vi "CombineVIScreenshots.vi"(6 "Image Types":T1[](array[typedef]), 8 "error in (no error)":errorcluster, 9 "Output Folders":T5, 10 "NewVI Screenshots in":T2, 11 "OldVI Screenshots in":T2) -> (0 "error out":errorcluster)   [LabVIEW 2015, in "VIDiffScreenshots.lvlib"]
uses:
  VIDiffScreenshots.lvlib
  Utilities/Output Folders.ctl
  VIScreenshots.ctl
  ScreenshotInfo.ctl
  Screenshot Type.ctl
  Utilities/FilePaths.ctl
  Utilities/VIDiffUtilities.lvlib
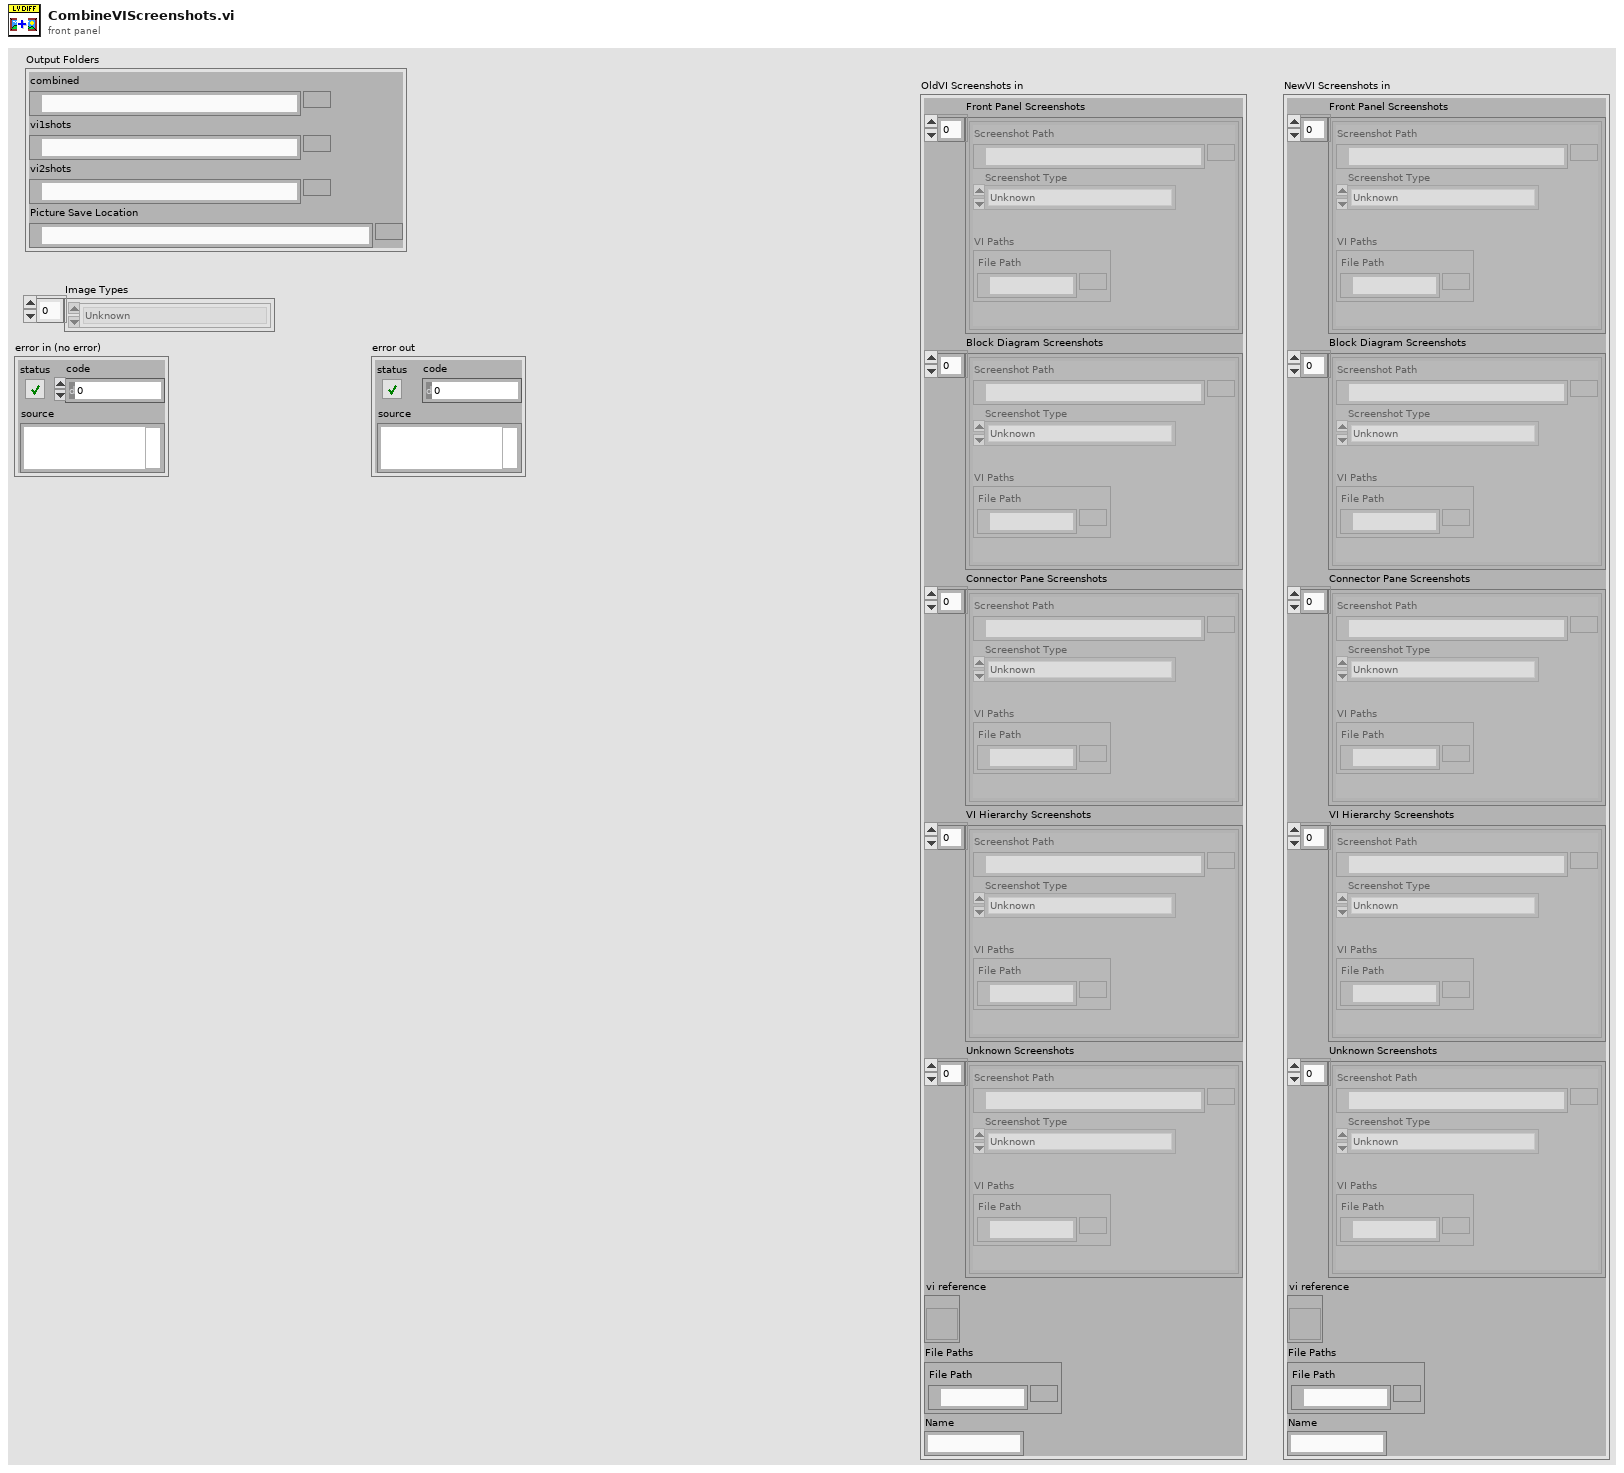
[diagram p1: front panel]
types:
  T1 = typedef "VIDiffScreenshots.lvlib/Screenshot Type.ctl" = enum16{"Unknown", "Front Panel", "Connector Pane", "Block Diagram", "VI Hierarchy"}
  T2 = typedef "VIDiffScreenshots.lvlib/VIScreenshots.ctl" = cluster{"Front Panel Screenshots":T3[], "Block Diagram Screenshots":T3[], "Connector Pane Screenshots":T3[], "VI Hierarchy Screenshots":T3[], "Unknown Screenshots":T3[], "vi reference":refnum<vi>, "File Paths":cluster{"File Path":path}, "Name":string}
  T3 = typedef "VIDiffScreenshots.lvlib/ScreenshotInfo.ctl" = cluster{"Screenshot Path":path, "Screenshot Type":T1, "VI Paths":T4}
  T4 = typedef "VIDiffUtilities.lvlib/FilePaths.ctl" = cluster{"File Path":path}
  T5 = typedef "VIDiffUtilities.lvlib/Output Folders.ctl" = cluster{"combined":path, "vi1shots":path, "vi2shots":path, "Picture Save Location":path}
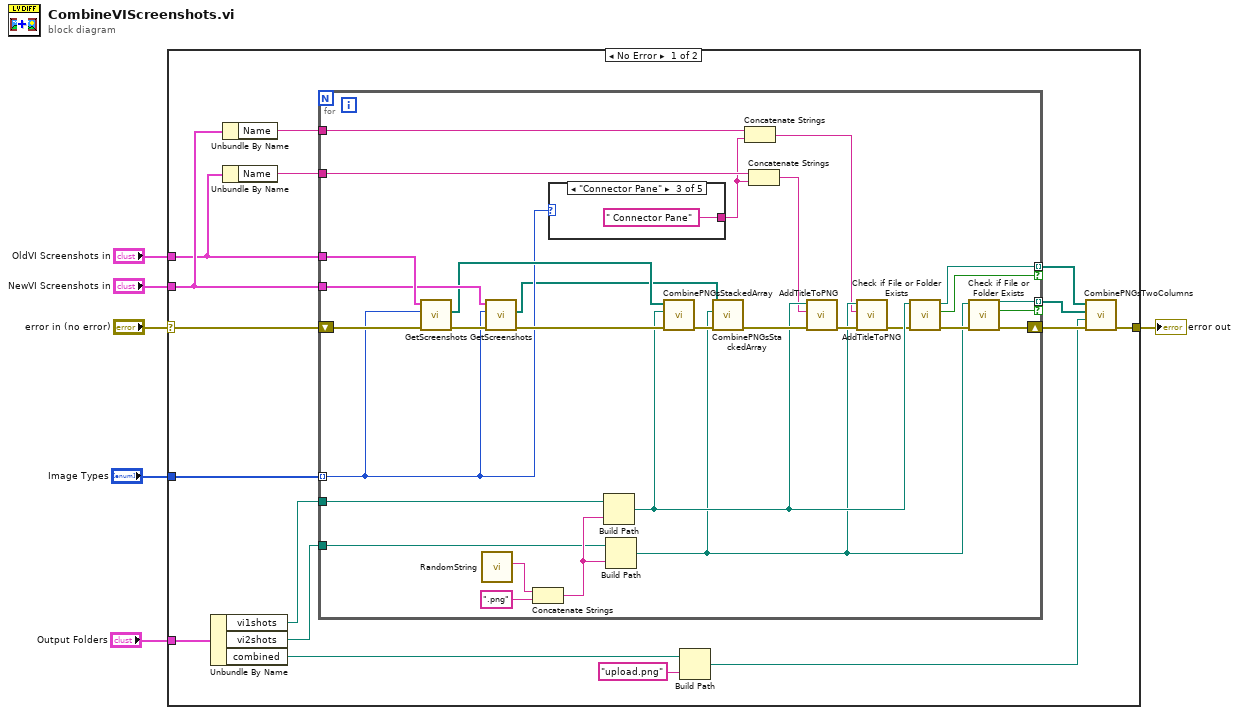
[diagram p0: block diagram]
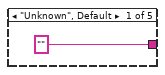
[diagram p2: hidden frame]
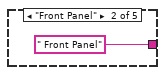
[diagram p3: hidden frame]
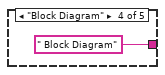
[diagram p4: hidden frame]
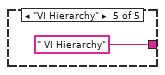
[diagram p5: hidden frame]
diagram:
  n1 = case shown="No Error" "error in (no error)" {
    selector: "error in (no error)" -> [w7 w58]
    tunnel: [w22 w58] -> w6
    tunnel: "Image Types" -> [w18 _]
    tunnel: "Output Folders" -> [w17 _]
    tunnel: "NewVI Screenshots in" -> [w10 _]
    tunnel: "OldVI Screenshots in" -> [w9 _]
    frame No Error {
      n2 = Unbundle By Name(w17) -> ("vi1shots"=w16:path, "vi2shots"=w15:path, "combined"=w13:path)
      n3 = Unbundle By Name(w10) -> ("Name"=w11:string)
      n4 = Unbundle By Name(w9) -> ("Name"=w8:string)
      n5 = for {
        shift-right: [w35] -> w19
        shift-left: w7 -> [w51]
        tunnel: w18 -> [w44] mode=indexing
        tunnel: w10 -> [w49]
        tunnel: w9 -> [w52]
        tunnel: w11 -> [w27]
        tunnel: [w33] -> w20 mode=indexing if=w32
        tunnel: [w31] -> w21 mode=indexing if=w30
        tunnel: w16 -> [w29]
        tunnel: w15 -> [w28]
        tunnel: w8 -> [w26]
        n6 = call "GetScreenshots.vi"("error in (no error)"=w51, "Screenshot Type"=w44, "VI Screenshots In"=w52) -> ("error out"=w50:errorcluster, "Screenshot Paths"=w48:path[])  [unwired: 7 in]
        n7 = call "RandomString.vi"() -> ("Random String"=w47:string)  [unwired: 11 in]
        n8 = call "GetScreenshots.vi"("error in (no error)"=w50, "Screenshot Type"=w44, "VI Screenshots In"=w49) -> ("error out"=w45:errorcluster, "Screenshot Paths"=w40:path[])  [unwired: 7 in]
        n9 = Concatenate Strings(w47, ".png" ("string")) -> (w41:string)
        n10 = case shown="\"Connector Pane\"" w44 {
          tunnel: ["" " Front Panel" " Connector Pane" " Block Diagram" " VI Hierarchy"] -> w23
          frame "Unknown", Default {
          }
          frame "Front Panel" {
          }
          frame "Connector Pane" {
          }
          frame "Block Diagram" {
          }
          frame "VI Hierarchy" {
          }
        }
        n11 = Build Path(base path=w29, name or relative path=w41) -> (appended path=w38:path)
        n12 = Build Path(base path=w28, name or relative path=w41) -> (appended path=w34:path)
        n13 = call "CombinePNGsStackedArray.vi"("error in (no error)"=w45, "Output File"=w38, "Input Files"=w48) -> ("error out"=w43:errorcluster)  [unwired: 8 in]
        n14 = call "CombinePNGsStackedArray.vi"("error in (no error)"=w43, "Output File"=w34, "Input Files"=w40) -> ("error out"=w42:errorcluster)  [unwired: 8 in]
        n15 = Concatenate Strings(w27, w23) -> (w24:string)
        n16 = Concatenate Strings(w26, w23) -> (w25:string)
        n17 = call "AddTitleToPNG.vi"("error in (no error)"=w42, "Title String"=w25, "PNG File"=w38) -> ("error out"=w39:errorcluster)  [unwired: 8 in]
        n18 = call "AddTitleToPNG.vi"("error in (no error)"=w39, "Title String"=w24, "PNG File"=w34) -> ("error out"=w37:errorcluster)  [unwired: 8 in]
        n19 = call <vilib>:"Check if File or Folder Exists.vi"("error in (no error)"=w37, "path"=w38) -> ("error out"=w36:errorcluster, "file or folder exists?"=w32:bool, "dup path"=w33:path)  [unwired: 7 in]
        n20 = call <vilib>:"Check if File or Folder Exists.vi"("error in (no error)"=w36, "path"=w34) -> ("error out"=w35:errorcluster, "file or folder exists?"=w30:bool, "dup path"=w31:path)  [unwired: 7 in]
      }
      n21 = Build Path(base path=w13, name or relative path="upload.png") -> (appended path=w12:path)
      n22 = call "CombinePNGsTwoColumns.vi"("error in (no error)"=w19, "Output File"=w12, "Right Column"=w21, "Left Column"=w20) -> ("error out"=w22:errorcluster)  [unwired: 7 in]
    }
    frame Error {
    }
  }
  "error out" <- w6
